vi "Detect Text.vi"   [LabVIEW 2020, in "feature_detection.lvlib" / "Text Detector.lvclass"]
uses:
  Text Detector.lvclass
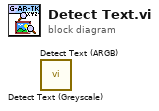
[diagram p0: block diagram]
diagram:
  n1 = call "Detect Text (Greyscale).vi"() -> ()  [unwired: 9 in, 3 out]
  n2 = call "Detect Text (ARGB).vi"() -> ()  [unwired: 9 in, 3 out]
